vi "SGL Array Registers.vi"(10 "SGL Array":sgl[](array[numeric]), 11 "I2C Register":T1) -> (3 "Data":u8[](array[numeric]))   [LabVIEW 2020, in "Rover.lvlib" / "Rover.lvclass"]
uses:
  Rover.lvclass
  I2C Register.ctl
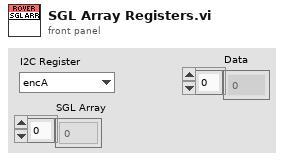
[diagram p1: front panel]
types:
  T1 = typedef "Rover.lvlib/Rover.lvclass/I2C Register.ctl" = enum8{"encA", "encB", "ticksPerUnit", "width", "flags", "velP", "velI", "velD", "velMin", "velMax", "poseX", "poseY", "poseA", "cmdDrive", "cmdTurn", "velocity", "turn", "velL", "velR", "run", "outL", "outR", "outDeadband"}
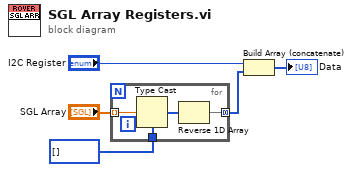
[diagram p0: block diagram]
diagram:
  n1 = for {
    tunnel: u8[] [] -> [w9]
    tunnel: "SGL Array" -> [w7] mode=indexing
    tunnel: [w6] -> w2 mode=concatenating
    n2 = Type Cast(type=w9, x=w7) -> (*(type *) &x=w8:u8[])
    n3 = Reverse 1D Array(array=w8) -> (reversed array=w6:u8[])
  }
  n4 = Build Array (concatenate)("I2C Register", w2) -> (→"Data":u8[])
